vi "Get Animations.vi"(8 "Error In":errorcluster, 11 "Display Manager In":refnum<class "Display Manager.lvclass">) -> (0 "Error Out":errorcluster, 2 "Animations":refnum<class "Animation.lvclass">[](array[class]), 3 "Display Manager Out":refnum<class "Display Manager.lvclass">)   [LabVIEW 2021, in "Display Manager.lvclass"]
uses:
  Display Manager.lvclass
  Display Manager.lvclass/Display Manager.ctl
  Animation/Animation.lvclass
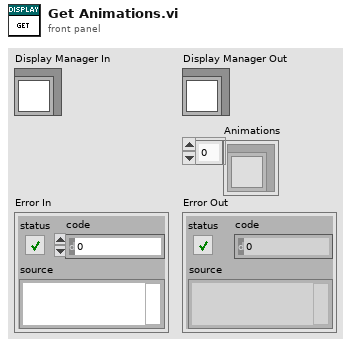
[diagram p1: front panel]
types:
  T1 = typedef "Display Manager.lvclass/Data.ctl" = cluster{"Size":T2, "Display Elements":refnum<class "Display Element.lvclass">[], "Frame":u32[][], "Animations":refnum<class "Animation.lvclass">[]}
  T2 = typedef "Display Utilities.lvlib/2D Dimensions.ctl" = cluster{"Width":i32, "Height":i32}
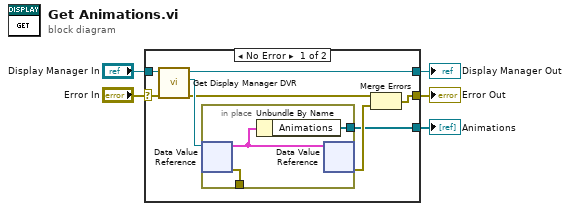
[diagram p0: block diagram]
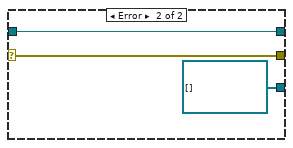
[diagram p2: hidden frame]
diagram:
  n1 = case shown="No Error" "Error In" {
    selector: "Error In" -> [w9 w18]
    tunnel: [w11 w18] -> w2
    tunnel: [w8 w19] -> w4
    tunnel: "Display Manager In" -> [w10 w19]
    tunnel: [w12 refnum<class "Animation.lvclass">[] [] ("Animations")] -> w1
    frame No Error {
      n2 = call "Get Display Manager DVR.vi"("Error In"=w9, "Display Manager In"=w10) -> ("Error Out"=w6:errorcluster, "DVR"=w7:refnum<data-value>, "Display Manager Out"=w8:refnum<class "Display Manager.lvclass">)  [unwired: 7 in]
      n3 = in-place {
        in-place-border: [w14] -> w12
        in-place-border: [w16] -> _
        n4 = in-place-dvr #1(w7) -> (w15:T1, w16:errorcluster)
        n5 = Unbundle By Name(w15) -> ("Animations"=w14:refnum<class "Animation.lvclass">[])
        n6 = in-place-dvr #1(w15) -> (w13:errorcluster)  [unwired: 1 out]
      }
      n7 = Merge Errors(w6, w13) -> (w11:errorcluster)
    }
    frame Error {
    }
  }
  "Display Manager Out" <- w4
  "Error Out" <- w2
  "Animations" <- w1
